vi "DrawGraph.vi"(7 "VI Refnum":refnum<vi>, 8 "error in (no error)":errorcluster, 11 "Array":waveform(dbl)[](array[waveform])) -> (0 "error out":errorcluster, 3 "file in tmp dir":path)   [LabVIEW 2018, in "TDMS_Word_Report.lvclass"]
uses:
  TDMS_Word_Report/TDMS_Word_Report.lvclass
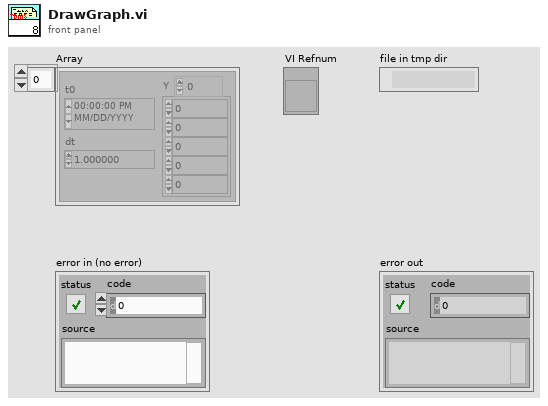
[diagram p1: front panel]
types:
  T1 = enum32{"Invalid", "Standard", "Closed", "Hidden", "Minimized", "Maximized"}
  T2 = typedef "imagedata.ctl" = cluster{"image type":i32, "image depth":i32, "image":u8[], "mask":u8[], "colors":u32[], "Rectangle":cluster{"left":i16, "top":i16, "right":i16, "bottom":i16}}
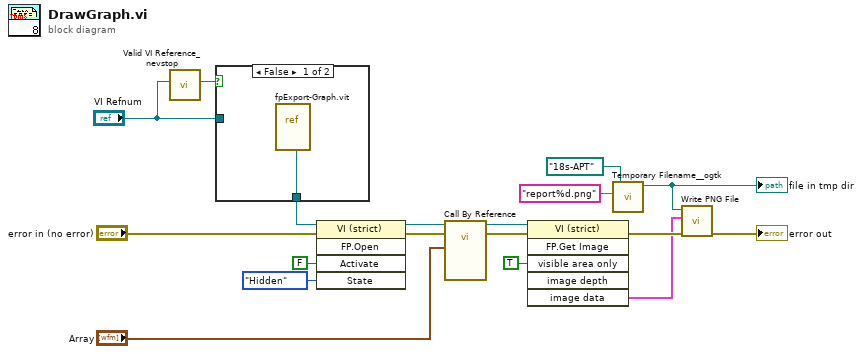
[diagram p0: block diagram]
diagram:
  n1 = call "Valid VI Reference_nevstop.vi"("VI Refnum"="VI Refnum") -> ("Valid?"=w2:bool)  [unwired: 9 in]
  n2 = case shown="False" w2 {
    tunnel: [w19 w20] -> w7
    tunnel: "VI Refnum" -> [_ w20]
    frame False {
      n3 = vi-ref "fpExport-Graph.vit"() -> (w19:refnum<vi>)
    }
    frame True {
    }
  }
  n4 = invoke on="Invoke Node" class="VI (strict)" method="FP.Open"(reference=w7, error in="error in (no error)", "Activate"=FALSE ("Activate?"), "State"=T1."Hidden") -> (reference out=w15:refnum<vi>, error out=w3:errorcluster)  [unwired: 1 in, 3 out]
  n5 = call-by-ref "Call By Reference"(reference=w15, error in=w3, "Waveform"="Array") -> (reference out=w9:refnum<vi>, error out=w8:errorcluster)  [unwired: 10 in, 1 out]
  n6 = invoke on="Invoke Node" class="VI (strict)" method="FP.Get Image"(reference=w9, error in=w8, "visible area only"=TRUE ("Visible Area Only")) -> (error out=w13:errorcluster, "image data"=w11:T2)  [unwired: 3 in, 4 out]
  n7 = call "Temporary Filename__ogtk.vi"("pattern (lvtemp%d.tmp)"="report%d.png", "sub directory"=path "18s-APT") -> ("file in tmp dir"=w12:path)  [unwired: 4 in, 1 out]
  "file in tmp dir" <- w12
  n8 = call <vilib>:"Write PNG File.vi"("error in (no error)"=w13, "image data"=w11, "path to PNG file"=w12) -> ("error out"=→"error out":errorcluster)  [unwired: 7 in, 1 out]
